vi "Construct Sink.vi"(9 "Error Action":T1=enum."Ignore Error and Close Sink", 10 "LogLevel":T2, 11 "ViewQueue":refnum<queue>) -> (3 "ConsoleSink out":refnum<class "ConsoleSink.lvclass">)   [LabVIEW 2017, in "ConsoleView.lvlib" / "ConsoleSink.lvclass"]
uses:
  ConsoleSink.lvclass
  C:/CS/Internal/LabVIEW/Logger/Source/Composed Log/Log Sink/Log Sink.lvclass
  Composed Log/Types/MessageCluster.ctl
  Composed Log/Types/Log Level.ctl
  Composed Log/Log Sink/Sink Error Actions ENUM.ctl
  ConsoleSink.lvclass/ConsoleSink.ctl
  Composed Log/Log Sink/Log Sink.lvclass/Log Sink.ctl
  Composed Log/Log Sink/Log Sink.lvclass
  Composed Log/Composed Log.lvlib
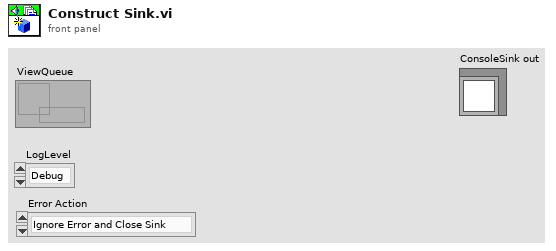
[diagram p1: front panel]
types:
  T1 = typedef "Composed Log.lvlib/Log Sink.lvclass/Sink Error Actions ENUM.ctl" = enum16{"Ignore Error and Continue", "Ignore Error and Close Sink", "Report Error and Close Sink"}
  T2 = typedef "Composed Log.lvlib/Log Level.ctl" = enum16{"Debug", "Info", "Warning", "Error", "Critical"}
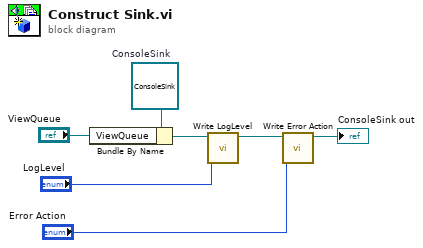
[diagram p0: block diagram]
diagram:
  w7 = refnum<class "ConsoleSink.lvclass"> refnum  # ConsoleSink
  n1 = Bundle By Name(cluster=w7, "ViewQueue"="ViewQueue") -> (w5:refnum<class "ConsoleSink.lvclass">)
  n2 = call "Write LogLevel.vi"("LogLevel"="LogLevel", "Log Sink in"=w5) -> ("Log Sink out"=w4:refnum<class "ConsoleSink.lvclass">)  [unwired: 8 in, 1 out]
  n3 = call "Write Error Action.vi"("Error Action"="Error Action", "Log Sink in"=w4) -> ("Log Sink out"=→"ConsoleSink out":refnum<class "ConsoleSink.lvclass">)  [unwired: 8 in, 1 out]
